vi "RescaleValue.vi"(0 "Old Scale Min":dbl, 1 "Old Scale Max":dbl, 2 "New Scale Min":dbl, 3 "New Scale Max":dbl, 4 "Input Value":dbl) -> (5 "Output Value":dbl)   [LabVIEW 2021]
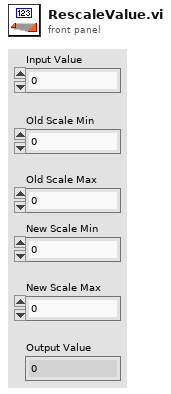
[diagram p1: front panel]
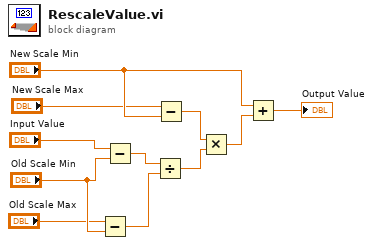
[diagram p0: block diagram]
diagram:
  n1 = Subtract(x="Old Scale Max", y="Old Scale Min") -> (x-y=w10:dbl)
  n2 = Subtract(x="Input Value", y="Old Scale Min") -> (x-y=w7:dbl)
  n3 = Divide(x=w7, y=w10) -> (x/y=w6:dbl)
  n4 = Subtract(x="New Scale Max", y="New Scale Min") -> (x-y=w3:dbl)
  n5 = Multiply(x=w3, y=w6) -> (x*y=w2:dbl)
  n6 = Add(x="New Scale Min", y=w2) -> (x+y=→"Output Value":dbl)
